vi "TurnToAngleController.vi"(0 "TargetAngle":dbl=600.0, 1 "MaxVel":dbl=80.0, 3 "MaxAccel":dbl=150.0, 5 "Robot":T1={"Angle"=548.1299999999924, "Angular vel"=0.49263510517714687, "Left Distance"=26.0882735, "Left vel"=0.0, "Right Distance"=-234.57467250000002, "Right vel"=0.0}, 9 "Gains":T2={"Gains"={"FFV"=0.0061, "FFA"=0.0024, "Vel PID"={"P"=0.0, "I"=0.0, "D"=0.0}}, "Pos PID"={"P"=0.0, "I"=0.0, "D"=0.0}, "MinVoltage"=0.25, "Effective Trackwidth CW"=30.0, "Effective Trackwidth CCW"=30.0} {"Pos PID"."D" format="%.3f"; "Pos PID"."I" format="%.3f"; "Pos PID"."P" format="%.3f"; "Gains"."Vel PID"."D" format="%.3f"; "Gains"."Vel PID"."I" format="%.3f"; "Gains"."Vel PID"."P" format="%.3f"}, 11 "Reset":bool) -> (4 "LeftPower":dbl=0.25, 6 "RightPower":dbl=-0.25, 8 "Encoder Distance":cluster{"Output":dbl, "dx/dt":dbl}(graph)={"Output"=52.36486996421861, "dx/dt"=26.0882735}, 10 "Delay":u32=20, 12 "Angle":cluster{"Distance":dbl, "CurrentAngle":dbl}(graph)={"Distance"=-120.0, "CurrentAngle"=-171.87000000000762}, 14 "VelGraph":cluster{"Output":dbl, "dx/dt":dbl}(graph), 15 "Done":bool)   [LabVIEW 2017]
uses:
  <vilib>/addons/control/pid/pid.llb/PID (DBL).vi
  <vilib>/addons/control/pid/NI_PID_pid.lvlib
panel:
  in  "Enable recalibrate":bool
  in  "GoSmallestDistance":bool
  in  "Target Vel":dbl
  out "Power":dbl(graph)=0.25
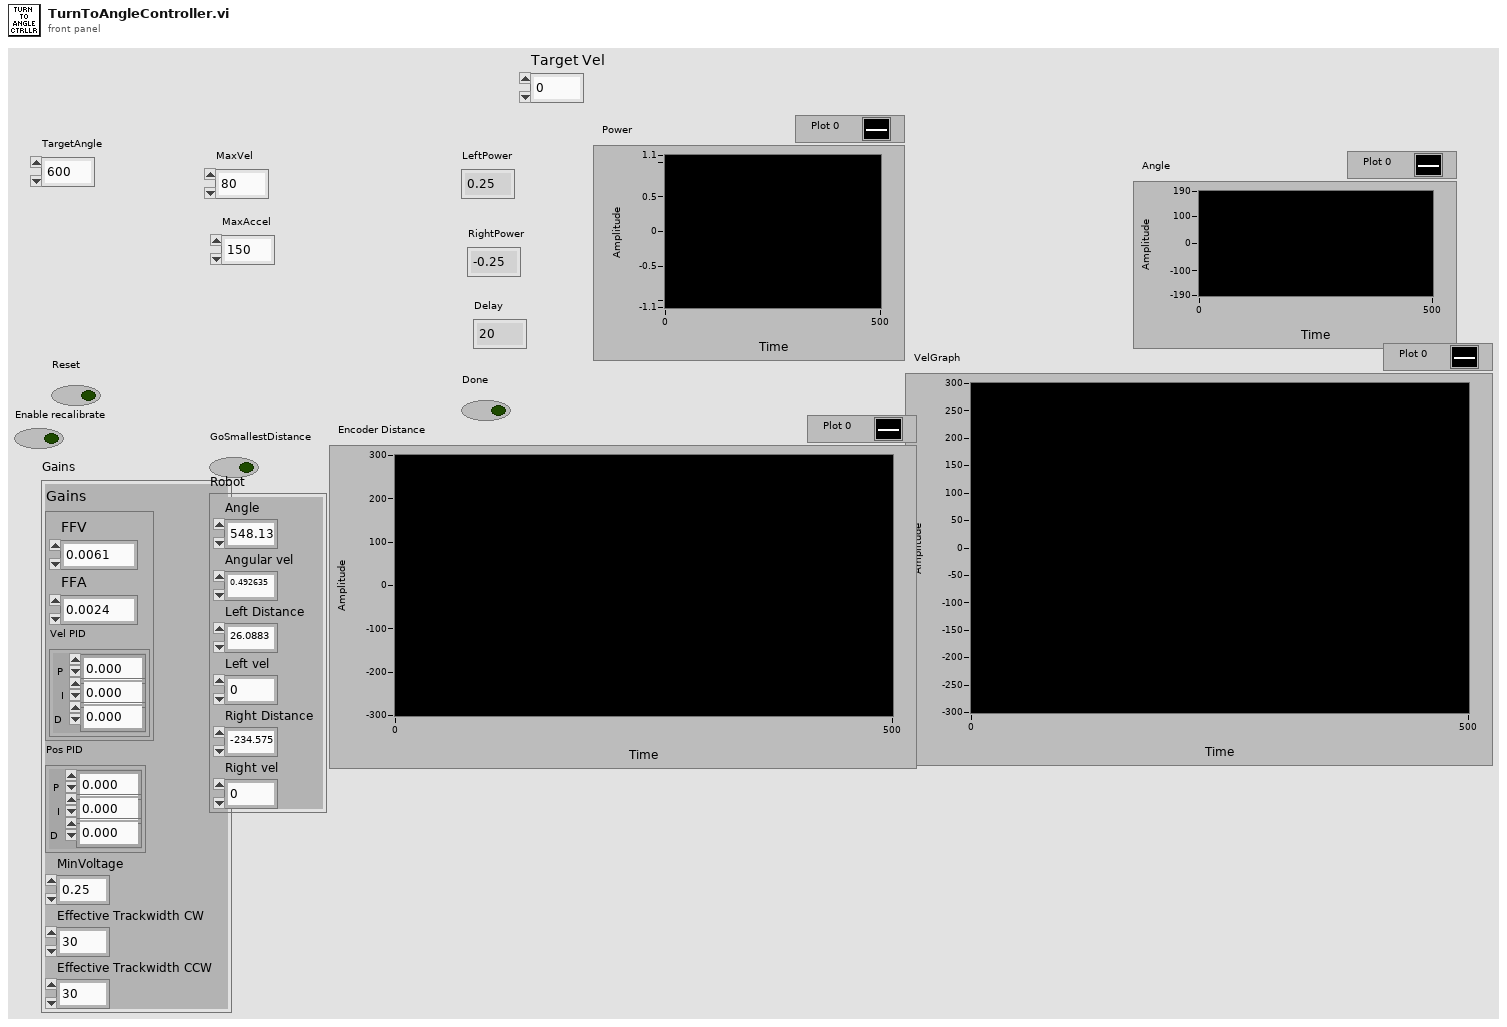
[diagram p1: front panel]
types:
  T1 = cluster{"Angle":dbl, "Angular vel":dbl, "Left Distance":dbl, "Left vel":dbl, "Right Distance":dbl, "Right vel":dbl}
  T2 = cluster{"Gains":cluster{"FFV":dbl, "FFA":dbl, "Vel PID":cluster{"P":dbl, "I":dbl, "D":dbl}}, "Pos PID":cluster{"P":dbl, "I":dbl, "D":dbl}, "MinVoltage":dbl, "Effective Trackwidth CW":dbl, "Effective Trackwidth CCW":dbl}
  T3 = cluster{"TargetPos":dbl, "InitalPos":dbl, "FinalVel":dbl, "IntitialVel":dbl, "MaxVel":dbl, "MaxAccel":dbl}
  T4 = cluster{"Smallest A to B":dbl, "Smallest A to B":dbl}
  T5 = cluster{"FFV":dbl, "FFA":dbl, "Vel PID":cluster{"P":dbl, "I":dbl, "D":dbl}}
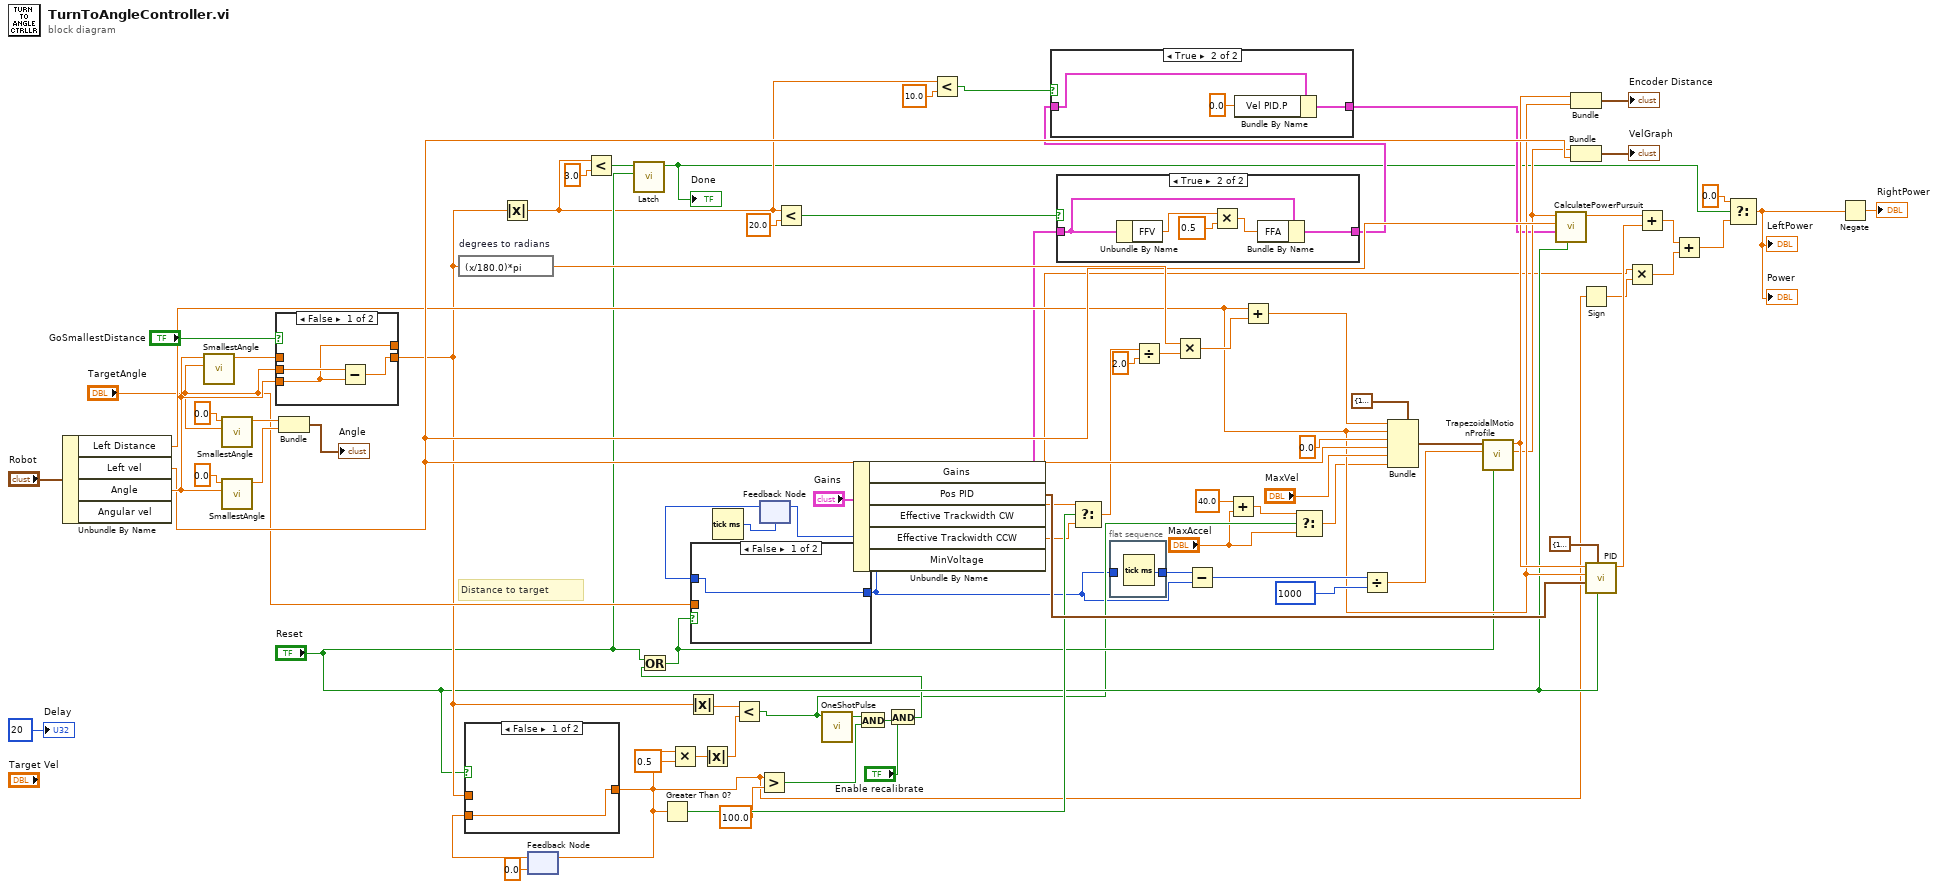
[diagram p0: block diagram]
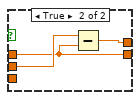
[diagram p5: hidden frame]
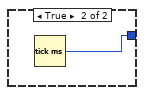
[diagram p6: hidden frame]
diagram:
  # "Distance to target"
  n1 = Unbundle By Name("Robot") -> ("Left Distance"=w47:dbl, "Left vel"=w52:dbl, "Angle"=w61:dbl)  [unwired: 1 out]
  n2 = call "SmallestAngle.vi"("Angle B"="TargetAngle", "Angle A"=w61) -> ("Smallest A to B"=w69:dbl)  [unwired: 9 in]
  n3 = call "SmallestAngle.vi"("Angle B"="TargetAngle", "Angle A"=0.0) -> ("Smallest A to B"=w59:dbl)  [unwired: 9 in]
  n4 = call "SmallestAngle.vi"("Angle B"=w61, "Angle A"=0.0) -> ("Smallest A to B"=w58:dbl)  [unwired: 9 in]
  n5 = case shown="False" "GoSmallestDistance" {
    tunnel: [w84 w88] -> _
    tunnel: "TargetAngle" -> [w85 w87]
    tunnel: w69 -> [_ w86]
    tunnel: [w83 w86] -> w34
    tunnel: w61 -> [w84 _]
    frame False {
      n6 = Subtract(x=w85, y=w84) -> (x-y=w83:dbl)
    }
    frame True {
      n7 = Subtract(x=w87, y=w86) -> (x-y=w88:dbl)
    }
  }
  n8 = Bundle("Smallest A to B"=w59, "Smallest A to B"=w58) -> (→"Angle":T4)  [unwired: 1 in]
  n9 = expression code="(x/180.0)*pi" "degrees to radians"(w34) -> (w55:dbl)
  n10 = Absolute Value(x=w34) -> (abs(x)=w21:dbl)
  n11 = feedback #1(0.0 ("Smallest A to B")) -> (w40:dbl)
  n12 = case shown="False" "Reset" {
    tunnel: w34 -> [_ w90]
    tunnel: [w89 w90] -> w2
    tunnel: w40 -> [w89 _]
    frame False {
    }
    frame True {
    }
  }
  n13 = feedback-in #1(w2) -> ()
  n14 = Less?(x=w21, y=3.0) -> (x < y?=w65:bool)
  n15 = call "Latch.vi"("Reset"="Reset", "Input"=w65) -> ("Output"=w1:bool)  [unwired: 9 in]
  "Done" <- w1
  n16 = Greater Than 0?(x=w2) -> (x > 0?=w38:bool)
  n17 = Multiply(x=w2, y=0.5) -> (x*y=w30:dbl)
  n18 = Absolute Value(x=w34) -> (abs(x)=w33:dbl)
  n19 = Absolute Value(x=w30) -> (abs(x)=w29:dbl)
  n20 = Tick Count (ms)() -> (millisecond timer value=w41:u32)
  n21 = Less?(x=w33, y=w29) -> (x < y?=w13:bool)
  n22 = Greater?(x=w2, y=100.0) -> (0:w14:bool)
  n23 = feedback #2(w41) -> (w42:u32)
  n24 = Less?(x=w21, y=20.0) -> (x < y?=w43:bool)
  n25 = call "OneShotPulse.vi"("Input"=w13) -> ("Output"=w17:bool)  [unwired: 10 in]
  n26 = Unbundle By Name("Gains") -> ("Gains"=w44:T5, "Pos PID"=w51:cluster{"P":dbl, "I":dbl, "D":dbl}, "Effective Trackwidth CW"=w37:dbl, "Effective Trackwidth CCW"=w36:dbl, "MinVoltage"=w3:dbl)
  n27 = And(x=w17, y=w14) -> (x .and. y?=w16:bool)
  n28 = And(x=w16, y="Enable recalibrate") -> (x .and. y?=w27:bool)
  n29 = Or(x="Reset", y=w27) -> (x .or. y?=w31:bool)
  n30 = case shown="False" w31 {
    tunnel: [w91 w92] -> w8
    tunnel: w42 -> [w91 _]
    tunnel: "TargetAngle" -> [_ _]
    frame False {
    }
    frame True {
      n31 = Tick Count (ms)() -> (millisecond timer value=w92:u32)
    }
  }
  n32 = feedback-in #2(w8) -> ()
  n33 = Less?(x=w21, y=10.0) -> (x < y?=w20:bool)
  n34 = case shown="True" w43 {
    tunnel: w44 -> [w93 w97]
    tunnel: [w93 w98] -> w19
    frame False {
    }
    frame True {
      n35 = Unbundle By Name(w97) -> ("FFV"=w96:dbl)
      n36 = Multiply(x=w96, y=0.5) -> (x*y=w94:dbl)
      n37 = Bundle By Name(cluster=w97, "FFA"=w94) -> (w98:T5)
    }
  }
  n38 = case shown="True" w20 {
    tunnel: w19 -> [w99 w101]
    tunnel: [w99 w102] -> w18
    frame False {
    }
    frame True {
      n39 = Bundle By Name(cluster=w101, "Vel PID.P"=0.0) -> (w102:T5)
    }
  }
  n40 = Select(t=w37, s=w38, f=w36) -> (s? t:f=w35:dbl)
  n41 = flat-sequence {
    tunnel: [w103] -> w75
    tunnel: w8 -> [_]
    frame #0 {
      n42 = Tick Count (ms)() -> (millisecond timer value=w103:u32)
    }
  }
  n43 = Divide(x=w35, y=2.0) -> (x/y=w56:dbl)
  n44 = Multiply(x=w55, y=w56) -> (x*y=w54:dbl)
  n45 = Subtract(x=w75, y=w8) -> (x-y=w74:u32)
  n46 = Add(x=40.0, y="MaxAccel") -> (x+y=w9:dbl)
  n47 = Add(x=w47, y=w54) -> (x+y=w53:dbl)
  n48 = Select(t=w9, s=w13, f="MaxAccel") -> (s? t:f=w11:dbl)
  n49 = Divide(x=w74, y=u32 1000) -> (x/y=w72:dbl)
  n50 = Bundle(cluster=T3 {"TargetPos"=10.0, "InitalPos"=0.0, "FinalVel"=0.0, "IntitialVel"=0.0, "MaxVel"=10.0, "MaxAccel"=10.0} ("Config"), "TargetPos"=w53, "InitalPos"=w47, "FinalVel"=0.0 ("IntitialVel"), "IntitialVel"=w52, "MaxVel"="MaxVel", "MaxAccel"=w11) -> (w76:T3)
  n51 = call "TrapezoidalMotionProfile.vi"("Initialize"=w31, "Time"=w72, "Config"=w76) -> ("Velocity"=w24:dbl, "Distance"=w49:dbl)  [unwired: 5 in, 2 out]
  n52 = call "CalculatePowerPursuit.vi"("Reset"="Reset", "Gains"=w18, "Vel"=w52, "Target Vel"=w24) -> ("Power"=w23:dbl)  [unwired: 7 in]
  n53 = Bundle("Distance"=w49, "Left Distance"=w47) -> (→"Encoder Distance":cluster{"Distance":dbl, "Left Distance":dbl})  [unwired: 1 in]
  n54 = Bundle("Velocity"=w24, "Left vel"=w52) -> (→"VelGraph":cluster{"Velocity":dbl, "Left vel":dbl})  [unwired: 1 in]
  n55 = Sign(1:w2) -> (0:w4:dbl)
  n56 = call-poly <vilib>:"PID.vi"("reinitialize? (F)"="Reset", "output range"=cluster{"output high":dbl, "output low":dbl} {"output high"=1.0, "output low"=-1.0}, "PID gains"=w51, "process variable"=w47, "setpoint"=w49) -> ("output"=w25:dbl)  [unwired: 5 in, 1 out]
  n57 = Multiply(x=w3, y=w4) -> (x*y=w5:dbl)
  n58 = Add(x=w23, y=w25) -> (x+y=w7:dbl)
  n59 = Add(x=w7, y=w5) -> (x+y=w6:dbl)
  n60 = Select(t=0.0, s=w1, f=w6) -> (s? t:f=w66:dbl)
  "LeftPower" <- w66
  "Power" <- w66
  n61 = Negate(x=w66) -> (-x=→"RightPower":dbl)
  "Delay" <- u32 20 ("Time Left")
